vi "readDataArray.vi"(8 "error in (no error)":errorcluster, 10 "array":string[][](array[string]), 11 "Dio64FileReader in":refnum<class "Dio64FileReader.lvclass">) -> (0 "error out":errorcluster, 3 "Dio64FileReader out":refnum<class "Dio64FileReader.lvclass">)   [LabVIEW 2011, in "Tools.lvlib" / "Filing.lvlib" / "Dio64FileReader.lvclass"]
uses:
  Dio64FileReader.lvclass
  Dio64FileReader.lvclass/Dio64FileReader.ctl
  Hal/Channels/Digital/DigitalOutput.lvclass
panel:
  out "data":dbl[][](array[numeric])
  out "Defaults":dbl[](array[numeric])
  out "channelAddresses":string[](array[string])
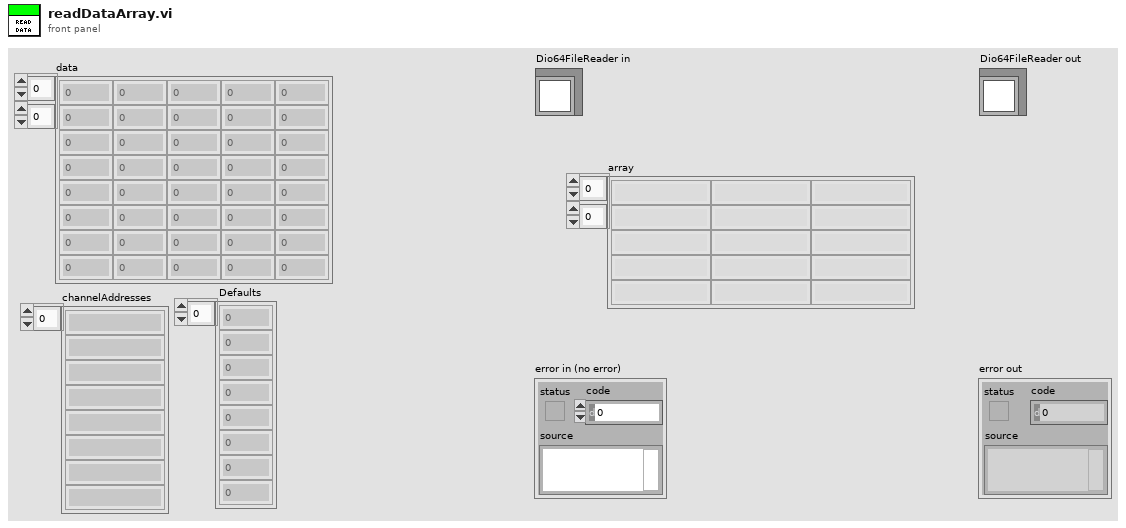
[diagram p1: front panel]
types:
  T1 = cluster{"Timestamps ms":dbl[], "DataPerChannel":dbl[][]}
  T2 = cluster{"Master Clock source":string, "Master Clock rate":dbl, "Start trigger line":string, "Scan rate":dbl, "Stop trigger line":string, "Sample Number":dbl}
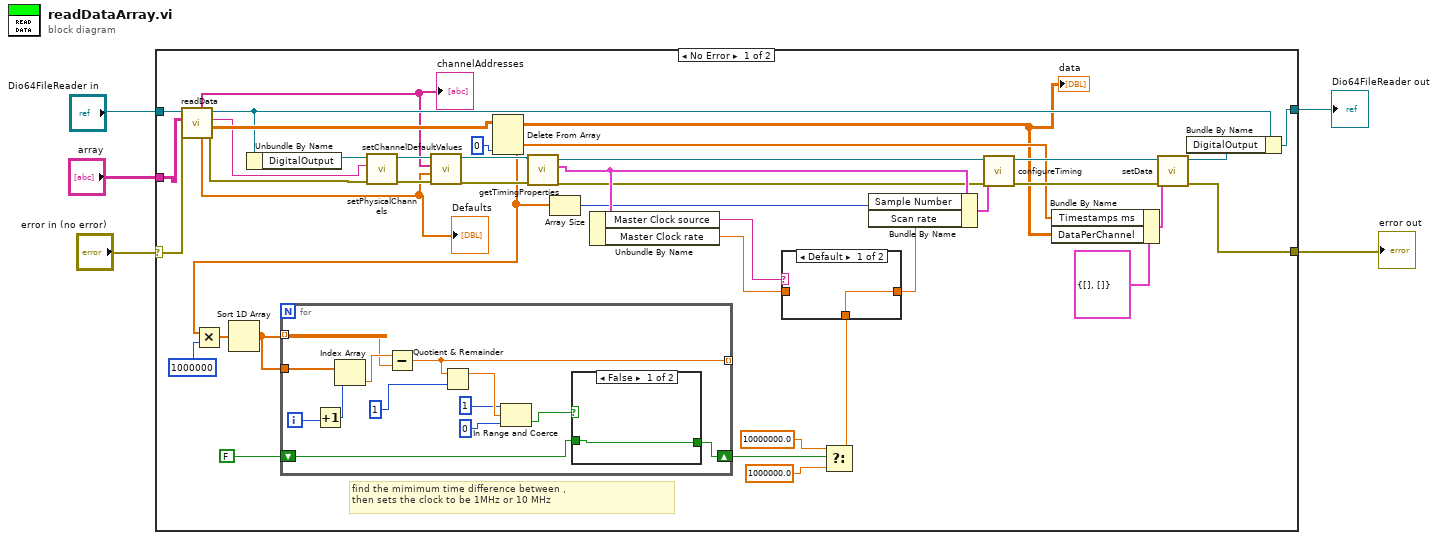
[diagram p0: block diagram]
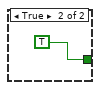
[diagram p3: hidden frame]
diagram:
  n1 = case shown="No Error" "error in (no error)" {
    selector: "error in (no error)" -> [w44 w63]
    tunnel: "Dio64FileReader in" -> [w45 w64]
    tunnel: [w29 w64] -> w2
    tunnel: [w8 w63] -> w1
    tunnel: "array" -> [w28 _]
    frame No Error {
      # "find the mimimum time difference between ,\nthen sets the clock to be 1MHz or 10 MHz"
      n2 = call-dynamic "readData.vi"("error in (no error)"=w44, "array"=w28, "FileReader in"=w45) -> ("error out"=w25:errorcluster, "Array"=w32:dbl[][], "channels"=w26:string, "FileReader out"=w30:refnum<class "Dio64FileReader.lvclass">, "Defaults"=w21:dbl[], "channelAddresses"=w22:string[])  [unwired: 3 in]
      "Defaults" <- w21
      "channelAddresses" <- w22
      n3 = Unbundle By Name(w30) -> ("DigitalOutput"=w27:refnum<class "DigitalOutput.lvclass">)
      n4 = call-dynamic "setPhysicalChannels.vi"("error in (no error)"=w25, "Physical Channels"=w26, "DigitalOutput.lvclass in"=w27) -> ("error out"=w23:errorcluster, "DigitalOutput.lvclass out"=w24:refnum<class "DigitalOutput.lvclass">)  [unwired: 7 in]
      n5 = call-dynamic "setChannelDefaultValues.vi"("error in (no error)"=w23, "calibratedValues"=w21, "channel_addresses"=w22, "DigitalOutput in"=w24) -> ("error out"=w18:errorcluster, "DigitalOutput out"=w19:refnum<class "DigitalOutput.lvclass">)  [unwired: 6 in]
      n6 = Delete From Array(array=w32, index (col)=0 ("disabled index (col)")) -> (deleted portion=w13:dbl[], array with subset deleted=w12:dbl[][])  [unwired: 2 in]
      "data" <- w12
      n7 = Multiply(x=w13, y=1000000) -> (x*y=w38:dbl[])
      n8 = Sort 1D Array(array=w38) -> (sorted array=w43:dbl[])
      n9 = for {
        tunnel: w43 -> [w56] mode=indexing
        tunnel: w43 -> [w60]
        tunnel: [w51] -> _ mode=indexing
        shift-right: [w48] -> w41
        shift-left: FALSE -> [w49]
        i -> [w59]
        n10 = Increment(x=w59) -> (x+1=w58:i32)
        n11 = Index Array(array=w60, index=w58) -> (element=w57:dbl)
        n12 = Subtract(x=w57, y=w56) -> (x-y=w51:dbl)
        n13 = Quotient & Remainder(x=w51, y=1) -> (x-y*floor(x/y)=w54:dbl)  [unwired: 1 out]
        n14 = In Range and Coerce(upper limit=1, x=w54, lower limit=0) -> (In Range?=w50:bool)  [unwired: 1 out]
        n15 = case shown="False" w50 {
          tunnel: w49 -> [w61 _]
          tunnel: [w61 TRUE] -> w48
          frame False {
          }
          frame True {
          }
        }
      }
      n16 = call-dynamic "getTimingProperties.vi"("error in (no error)"=w18, "DigitalOutput.lvclass in"=w19) -> ("error out"=w11:errorcluster, "Timing"=w20:T2, "DigitalOutput.lvclass out"=w9:refnum<class "DigitalOutput.lvclass">)  [unwired: 7 in]
      n17 = Array Size(array=w13) -> (size(s)=w6:i32)
      n18 = Unbundle By Name(w20) -> ("Master Clock source"=w36:string, "Master Clock rate"=w34:dbl)
      n19 = Select(t=10000000.0, s=w41, f=1000000.0) -> (s? t:f=w35:dbl)
      n20 = case shown="Default" w36 {
        tunnel: w35 -> [w46 _]
        tunnel: w34 -> [_ w47]
        tunnel: [w46 w47] -> w33
        frame Default {
        }
        frame "internal", "none" {
        }
      }
      n21 = Bundle By Name(cluster=w20, "Sample Number"=w6, "Scan rate"=w33) -> (w10:T2)
      n22 = call-dynamic "configureTiming.vi"("error in (no error)"=w11, "Timing"=w10, "DigitalOutput in"=w9) -> ("error out"=w17:errorcluster, "DigitalOutput out"=w16:refnum<class "DigitalOutput.lvclass">)  [unwired: 7 in]
      n23 = Bundle By Name(cluster=T1 {"Timestamps ms"=[], "DataPerChannel"=[]} ("Data"), "Timestamps ms"=w13, "DataPerChannel"=w12) -> (w14:T1)
      n24 = call-dynamic "setData.vi"("error in (no error)"=w17, "Data"=w14, "DigitalOutput.lvclass in"=w16) -> ("error out"=w8:errorcluster, "DigitalOutput.lvclass out"=w7:refnum<class "DigitalOutput.lvclass">)  [unwired: 7 in]
      n25 = Bundle By Name(cluster=w30, "DigitalOutput"=w7) -> (w29:refnum<class "Dio64FileReader.lvclass">)
    }
    frame Error {
    }
  }
  "error out" <- w1
  "Dio64FileReader out" <- w2
